vi "New SenseHat.vi"(8 "error in (no error)":errorcluster, 11 "LINX Resource":T1={"IO"=enum."Remote", "Interface"=enum."Serial", "LINX Device Config"={"Interface"=enum."Serial", "COM Port"="COM13", "TCP Configuration"={"IP Address"="", "Port"=0}, "Device Family"=1, "Device ID"=1, "Device Name"="myRIO-1900", "TCP Ref"=refnum, "Channels"={"DI"=[0, 1, 2, 3, 4, 5, 6, 7, 8, 9, 10, 11, 12, 13, 14, 15, 16, 17, 18, 19, 20, 21, 22, 23, 24, 25, 26, 27, 28, 29, 30, 31, 32, 33, 34, 35, 36, 37, 38, 39, 40, 41, 42, 43, 44, 45, 46], "DO"=[0, 1, 2, 3, 4, 5, 6, 7, 8, 9, 10, 11, 12, 13, 14, 15, 16, 17, 18, 19, 20, 21, 22, 23, 24, 25, 26, 27, 28, 29, 30, 31, 32, 33, 34, 35, 36, 37, 38, 39, 40, 41, 42, 43, 44, 45, 46], "AI"=[0, 1, 2, 3, 4, 5, 6, 7, 8, 9, 10, 11], "AO"=[], "PWM"=[3, 5, 6, 9, 10], "QE"=[], "UART"=[0, 1], "I2C 2"=[0], "SPI"=[0], "CAN"=[], "Servo"=[], "AI Ref (V)"=0.0, "AI Resolution (Bits)"=0, "AO Ref (V)"=0.0, "AO Resolution (Bits)"=0}}}) -> (0 "error out":errorcluster, 3 "LINX-SenseHat out":refnum<class "LINX-SenseHat.lvclass">)   [LabVIEW 2020, in "LINX-SenseHat.lvclass"]
doc: "Creates a new sense-hat reference from the configured LINX reference."
uses:
  LINX-SenseHat.lvclass
  <vilib>/MakerHub/LINX/Private/Type Defs/LINX Ref.ctl
  <vilib>/MakerHub/LINX/Private/Type Defs/Platform.ctl
  <vilib>/MakerHub/LINX/Private/Type Defs/Interface.ctl
  <vilib>/MakerHub/LINX/Private/Device/Type Defs/LINX Device Config.ctl
  <vilib>/MakerHub/LINX/Private/Device/Type Defs/TCP Config.ctl
  <vilib>/MakerHub/LINX/Private/Device/Type Defs/Channels.ctl
  HTS221/HTS221 Data Rates.ctl
  LINX-SenseHat.lvclass/LINX-SenseHat.ctl
  LINX I2C/LINX I2C.lvclass
  LPS Barometric Pressure/LPS Barometric Pressure Sensor.lvclass
  HTS221/HTS221.lvclass
  LSM9DS1/LSM9DS1 IMU.lvclass
  <vilib>/MakerHub/LINX/LMH-LINX.lvlib
  <vilib>/MakerHub/LINX/Private/Device/Device.lvlib
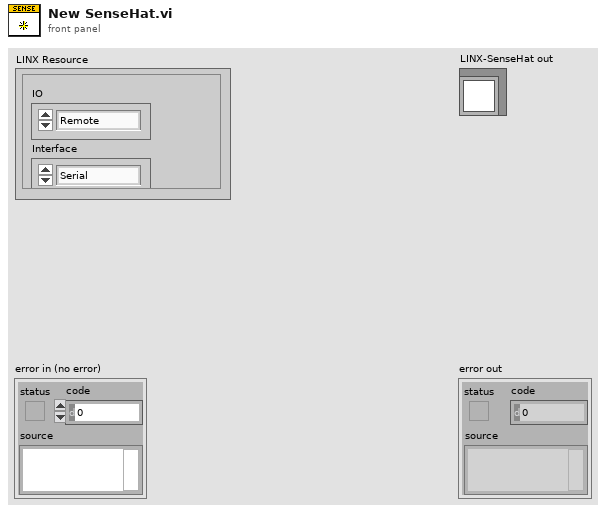
[diagram p1: front panel]
types:
  T1 = typedef "LMH-LINX.lvlib/LINX Ref.ctl" = cluster{"IO":T2, "Interface":T3, "LINX Device Config":T4}
  T2 = typedef "LMH-LINX.lvlib/Platform.ctl" = enum16{"Remote", "Local"}
  T3 = typedef "LMH-LINX.lvlib/Interface.ctl" = enum16{"Serial", "TCP"}
  T4 = typedef "LMH-LINX.lvlib/Device.lvlib/LINX Device Config.ctl" = cluster{"Interface":T3, "COM Port":refnum<visa-resource-name>, "TCP Configuration":T5, "Device Family":u8, "Device ID":u8, "Device Name":string, "TCP Ref":refnum<k5>, "Channels":T6}
  T5 = typedef "LMH-LINX.lvlib/Device.lvlib/TCP Config.ctl" = cluster{"IP Address":string, "Port":u16}
  T6 = typedef "LMH-LINX.lvlib/Channels.ctl" = cluster{"DI":u8[], "DO":u8[], "AI":u8[], "AO":u8[], "PWM":u8[], "QE":u8[], "UART":u8[], "I2C 2":u8[], "SPI":u8[], "CAN":u8[], "Servo":u8[], "AI Ref (V)":dbl, "AI Resolution (Bits)":u8, "AO Ref (V)":dbl, "AO Resolution (Bits)":u8}
  T7 = typedef "HTS221.lvclass/HTS221 Data Rates.ctl" = enum16{"One-Shot", "1Hz", "7Hz", "12.5Hz"}
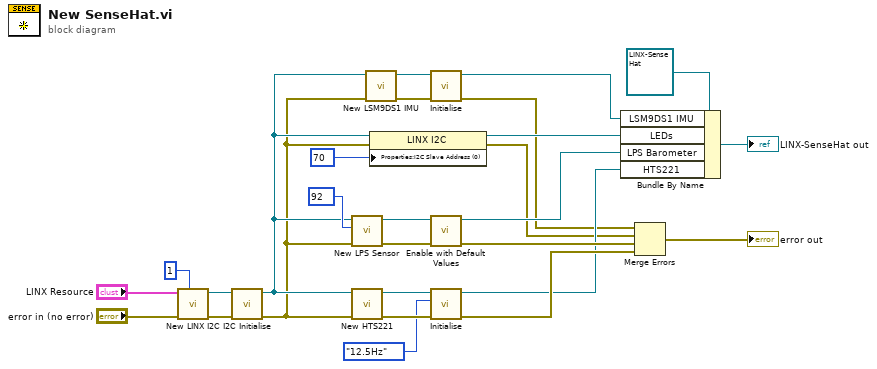
[diagram p0: block diagram]
diagram:
  n1 = call "New LINX I2C.vi"("LINX I2C Channel"=u8 1, "error in (no error)"="error in (no error)", "LINX Resource"="LINX Resource") -> ("error out"=w12:errorcluster, "LINX I2C out"=w14:refnum<class "LINX I2C.lvclass">)  [unwired: 7 in]
  n2 = call-dynamic "I2C Initialise.vi"("error in (no error)"=w12, "LINX I2C in"=w14) -> ("error out"=w5:errorcluster, "LINX I2C out"=w6:refnum<class "LINX I2C.lvclass">)  [unwired: 8 in]
  n3 = call "New LPS Sensor.vi"("error in (no error)"=w5, "I2C Slave Address (0x5D)"=u8 92, "I2C"=w6) -> ("error out"=w27:errorcluster, "LPS Barometer out"=w26:refnum<class "LPS Barometric Pressure Sensor.lvclass">)  [unwired: 7 in]
  n4 = call "New HTS221.vi"("error in (no error)"=w5, "I2C in"=w6) -> ("error out"=w25:errorcluster, "HTS221 out"=w24:refnum<class "HTS221.lvclass">)  [unwired: 8 in]
  n5 = call "New LSM9DS1 IMU.vi"("error in (no error)"=w5, "I2C in"=w6) -> ("error out"=w4:errorcluster, "LSM9DS1 IMU out"=w3:refnum<class "LSM9DS1 IMU.lvclass">)  [unwired: 8 in]
  n6 = property class="LINX I2C"(reference=w6, error in=w5, "Properties:I2C Slave Address (0)"=u8 70 ("I2C Slave Address (0x5D)")) -> (reference out=w8:refnum<class "LINX I2C.lvclass">, error out=w9:errorcluster)
  n7 = call "Initialise.vi"("error in (no error)"=w4, "LSM9DS1 IMU in"=w3) -> ("error out"=w2:errorcluster, "LSM9DS1 IMU out"=w1:refnum<class "LSM9DS1 IMU.lvclass">)  [unwired: 8 in]
  n8 = call-dynamic "Enable with Default Values.vi"("error in (no error)"=w27, "LPS Barometer in"=w26) -> ("error out"=w22:errorcluster, "LPS Barometer out"=w18:refnum<class "LPS Barometric Pressure Sensor.lvclass">)  [unwired: 8 in]
  n9 = call "Initialise.vi"("error in (no error)"=w25, "Data Rate (12.5Hz)"=HTS221_Data_Rates."12.5Hz", "HTS221 in"=w24) -> ("error out"=w23:errorcluster, "HTS221 out"=w17:refnum<class "HTS221.lvclass">)  [unwired: 7 in]
  n10 = Bundle By Name(cluster=refnum<class "LINX-SenseHat.lvclass"> refnum ("LINX-SenseHat out"), "LSM9DS1 IMU"=w1, "LEDs"=w8, "LPS Barometer"=w18, "HTS221"=w17) -> (→"LINX-SenseHat out":refnum<class "LINX-SenseHat.lvclass">)
  n11 = Merge Errors(w2, w9, w22, w23) -> (→"error out":errorcluster)
